vi "Up Hole PRESSURE_CAL 2016.vi"(1 "Zero Pressure\n(F = leave as is)":bool=TRUE, 4 "Pressure \nOffset\nInput":dbl=24.27199935913086 format="%.2f", 6 "Descriptions":string[](array[string]), 7 "Array in":refnum<k24>[](array[refnum]), 9 "Pressure \nSlope\nInput":dbl=24.27199935913086 format="%.2f", 10 "Sensor Cluster":T1, 11 "Prompt_IN":string) -> (2 "Pressure \nOffset FG\nOutput":dbl=24.27199935913086 format="%.2f", 3 "PRESSURE\nFt of water":dbl format="%.2f", 5 "Array out":refnum<k24>[](array[refnum]))   [LabVIEW 2016]
uses:
  controls/MCC DAQ Readings.ctl
  C:/Cascade-lv16-64/builds/Waterloo Main Program/cascade/data/ULx_LV.dll
  builds/Waterloo Main Program/cascade/data/ULx_LV.dll
  Kpro Globals.vi
panel:
  out "Loop Counter":i32
  out "Setup_instructions":string
  in  "OK Button":bool
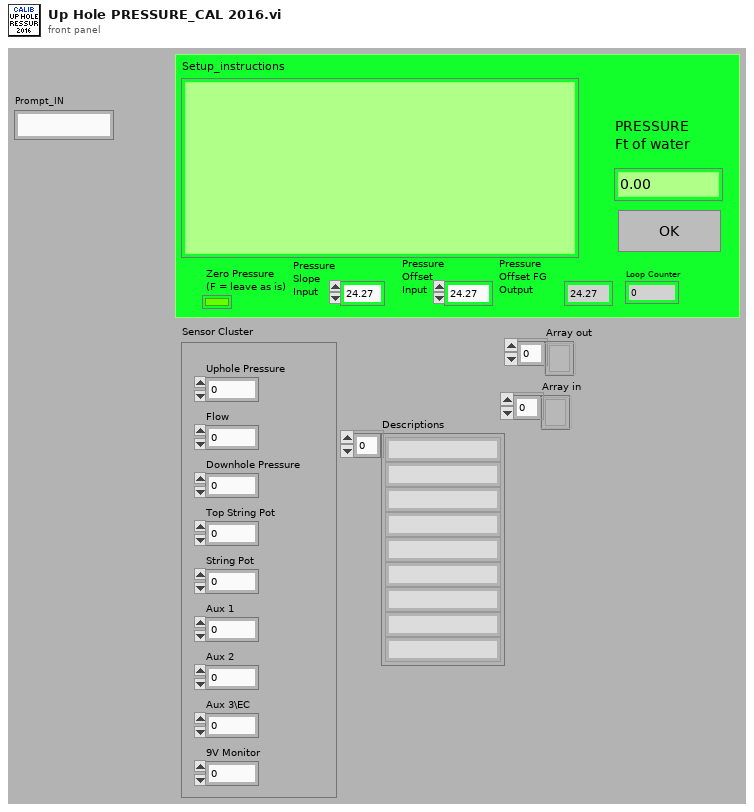
[diagram p1: front panel]
types:
  T1 = typedef "MCC DAQ Readings.ctl" = cluster{"Uphole Pressure":dbl, "Flow":dbl, "Downhole Pressure":dbl, "Top String Pot":dbl, "String Pot":dbl, "Aux 1":dbl, "Aux 2":dbl, "Aux 3\\EC":dbl, "9V Monitor":dbl}
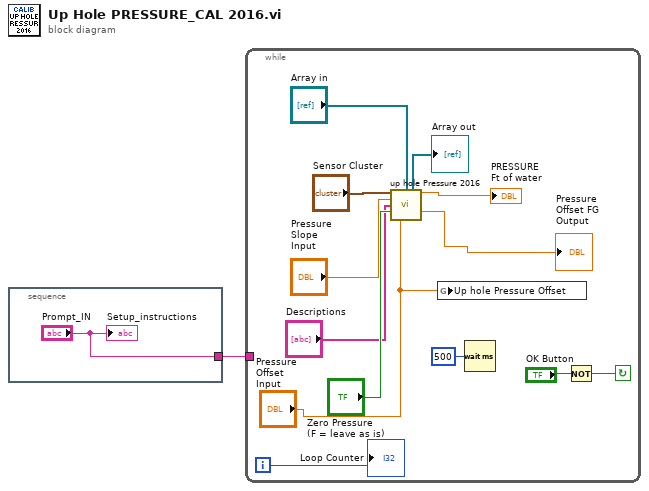
[diagram p0: block diagram]
diagram:
  n1 = stacked-sequence {
    tunnel: ["Prompt_IN"] -> w1
    frame #0 {
      "Setup_instructions" <- "Prompt_IN"
    }
  }
  n2 = while {
    tunnel: w1 -> [_]
    i -> [w5]
    stop <- w13 continue-if-true
    n3 = call "up hole Pressure 2016.vi"("Sensor Cluster"="Sensor Cluster", "Up Hole Pressure\n Offset Input"="Pressure \nOffset\nInput", "Array in"="Array in", "Pressure \nSlope"="Pressure \nSlope\nInput", "Descriptions"="Descriptions", "Zero Pressure\n(F = leave as is)"="Zero Pressure\n(F = leave as is)") -> ("Array out"=→"Array out":refnum<k24>[], "Uphole Pressure"=→"PRESSURE\nFt of water":dbl, "Uphole Pressure FG Offset Output"=→"Pressure \nOffset FG\nOutput":dbl)  [unwired: 6 in, 1 out]
    n4 = global write "Kpro Globals.vi" "Up hole Pressure Offset"("Pressure \nOffset\nInput") -> ()
    n5 = Wait (ms)(milliseconds to wait=u32 500) -> ()  [unwired: 1 out]
    n6 = Not(x="OK Button") -> (.not. x?=w13:bool)
    "Loop Counter" <- w5
  }
